vi "NI VeriStand - Set Log File Producer Flag.vi"(8 "error in (no error)":errorcluster, 10 "Log File Producer":bool, 11 "Item Ref in":T1 format="%.0x") -> (0 "error out":errorcluster, 3 "Item Ref out":T1 format="%.0x")   [LabVIEW 2020, in "Custom Device API.lvlib"]
doc: "Sets a property for the specified custom device item that indicates whether the item produces log files. When TRUE, you can use the Data Logging control to download log files produced by the item."
uses:
  <vilib>/NI VeriStand/Custom Device API/Custom Device API.lvlib
  <vilib>/NI VeriStand/Custom Device API/Custom Device Item Ref.ctl
  75958f06-e5d4-4e19-98cb-b9f5729aeb3c.vi
  <vilib>/NI VeriStand/Custom Device API/Custom Device Offline Path.vi
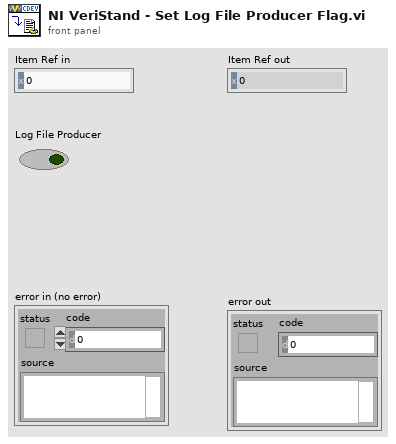
[diagram p1: front panel]
types:
  T1 = typedef "Custom Device API.lvlib/Custom Device Item Ref.ctl" = u64
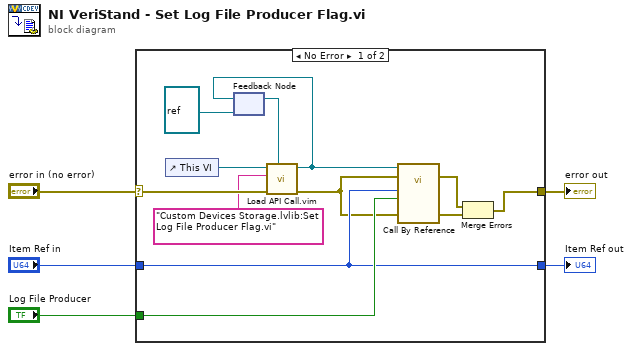
[diagram p0: block diagram]
diagram:
  n1 = case shown="No Error" "error in (no error)" {
    selector: "error in (no error)" -> [w11 w19]
    tunnel: [w17 w19] -> w5
    tunnel: "Item Ref in" -> [w14 w18]
    tunnel: "Log File Producer" -> [w15 _]
    tunnel: [w14 w18] -> w1
    frame No Error {
      n2 = control-ref of="This VI"() -> (w12:refnum<vi>)
      n3 = feedback #1(refnum<vi> refnum ("type specifier VI Refnum (for type only)")) -> (w13:refnum<vi>)
      n4 = call "Load API Call.vim"("VI reference in"=w13, "error in (no error)"=w11, "VI qualified name"="Custom Devices Storage.lvlib:Set Log File Producer Flag.vi", "Caller VI ref"=w12) -> ("error out"=w10:errorcluster, "VI reference"=w9:refnum<vi>)  [unwired: 6 in]
      n5 = feedback-in #1(w9) -> ()
      n6 = call-by-ref "?"(reference=w9, error in=w10, 8:"error in (no error)"=w10, "Log File Provider"=w15, "Item Ref in"=w14) -> (error out=w6:errorcluster, 0:"error out"=w16:errorcluster)  [unwired: 8 in, 1 out]
      n7 = Merge Errors(w6, w16) -> (w17:errorcluster)
    }
    frame Error {
    }
  }
  "Item Ref out" <- w1
  "error out" <- w5
